vi "S4GUI_003.vi"(7 "Tab ObsEng":enum32{"Obs", "CCD modes", "Guider", "Eng"}(tab)) -> ()   [LabVIEW 2018] (continued)
            n1724 = call-dynamic "Write State Machine.vi"("error in (no error)"=w3191, "State Machine.lvclass"=w3193, "Device in"=w3195) -> ("error out"=w3188:errorcluster, "Device out"=w3189:refnum<class "Channel.lvclass">)  [unwired: 7 in]
            n1725 = call-dynamic "Write Channel.vi"("error in (no error)"=w3188, "Channel.lvclass"=w3189, "Acquisition in"=w3197) -> ("error out"=w3187:errorcluster, "Acquisition out"=w3186:refnum<class "Acquisition.lvclass">)  [unwired: 7 in]
            n1726 = call-dynamic "Write AcquisitionC.vi"("error in (no error)"=w3187, "Acquisition.lvclass"=w3186, "S4ACS_GUI in"=w3199) -> ("error out"=w3157:errorcluster, "S4ACS_GUI out"=w3156:refnum<class "S4GUI.lvclass">)  [unwired: 7 in]
            n1727 = call-dynamic "Read AcquisitionD.vi"("error in (no error)"=w3157, "S4ACS_GUI in"=w3156) -> ("error out"=w3165:errorcluster, "Acquisition.lvclass"=w3163:refnum<class "Acquisition.lvclass">, "S4ACS_GUI out"=w3162:refnum<class "S4GUI.lvclass">)  [unwired: 7 in]
            n1728 = call-dynamic "Read Channel.vi"("error in (no error)"=w3165, "Acquisition in"=w3163) -> ("error out"=w3178:errorcluster, "Channel.lvclass"=w3176:refnum<class "Channel.lvclass">, "Acquisition out"=w3164:refnum<class "Acquisition.lvclass">)  [unwired: 7 in]
            n1729 = call "Write section_name.vi"("error in (no error)"=w3178, "section_name"="CCD_ACS4", "Channel in"=w3176) -> ("error out"=w3179:errorcluster, "Channel out"=w3177:refnum<class "Channel.lvclass">)  [unwired: 7 in]
            n1730 = call-dynamic "load config.vi"("error in (no error)"=w3179, "cfg file name"=w3150, "Channel in"=w3177) -> ("error out"=w3136:errorcluster, "Channel out"=w3134:refnum<class "Channel.lvclass">)  [unwired: 7 in]
            n1731 = call-dynamic "save config.vi"("error in (no error)"=w3136, "file config"="lastsaved.cfg", "Channel in"=w3134) -> ("error out"=w3135:errorcluster, "Channel out"=w3133:refnum<class "Channel.lvclass">)  [unwired: 7 in]
            n1732 = call-dynamic "Read State Machine.vi"("error in (no error)"=w3135, "Device in"=w3133) -> ("error out"=w3169:errorcluster, "State Machine.lvclass"=w3167:refnum<class "State Machine.lvclass">, "Device out"=w3166:refnum<class "Channel.lvclass">)  [unwired: 7 in]
            n1733 = call-dynamic "Write State.vi"("error in (no error)"=w3169, "State"=60, "State Machine in"=w3167) -> ("error out"=w3170:errorcluster, "State Machine out"=w3168:refnum<class "State Machine.lvclass">)  [unwired: 7 in]
            n1734 = call-dynamic "Write State Machine.vi"("error in (no error)"=w3170, "State Machine.lvclass"=w3168, "Device in"=w3166) -> ("error out"=w3173:errorcluster, "Device out"=w3172:refnum<class "Channel.lvclass">)  [unwired: 7 in]
            n1735 = call-dynamic "Write Channel.vi"("error in (no error)"=w3173, "Channel.lvclass"=w3172, "Acquisition in"=w3164) -> ("error out"=w3174:errorcluster, "Acquisition out"=w3175:refnum<class "Acquisition.lvclass">)  [unwired: 7 in]
            n1736 = call-dynamic "Write AcquisitionD.vi"("error in (no error)"=w3174, "Acquisition.lvclass"=w3175, "S4ACS_GUI in"=w3162) -> ("error out"=w3153:errorcluster, "S4ACS_GUI out"=w3155:refnum<class "S4GUI.lvclass">)  [unwired: 7 in]
            n1737 = Unbundle By Name(w3106) -> ("INITIAL_LINE"=w3127:u16, "INITIAL_COLUMN"=w3126:u16, "FINAL_LINE"=w3125:u16, "FINAL_COLUMN"=w3124:u16, "VBIN"=w3123:u16, "HBIN"=w3122:u16, "PREAMP"=w3121:u8, "EM_GAIN"=w3120:u16, "READOUT_RATE"=w3119:u8, "SHUTTER_OPENING_TIME"=w3118:u16, "SHUTTER_CLOSING_TIME"=w3117:u16, "VERTICAL_SHIFT_SPEED"=w3107:u8, "READ_MODE"=w3116:u8, "VERTICAL_CLOCK_VOLTAGE"=w3115:u8, "AD_CHANNEL"=w3114:u32, "SHUTTER_MODE"=w3113:u8, "SHUTTER_TTL"=w3112:u8, "TRIGGER_MODE"=w3111:u8, "FRAME_TRANSFER"=w3110:bool, "ACQUISITION_MODE"=w3109:u8, "EM_MODE"=w3108:u8)
            n1738 = call "Write cfg file.vi"("error in (no error)"=w3153, "cfg file"=w3150, "S4ACS_GUI in"=w3155) -> ("error out"=w3152:errorcluster, "S4ACS_GUI out"=w3154:refnum<class "S4GUI.lvclass">)  [unwired: 7 in]
            n1739 = local read "Input Cluster"() -> (w3129:T8)
            n1740 = Bundle By Name(cluster=w3129, "Parameters.Image \nInitial Line"=w3127, "Parameters.Image\nInitial Column"=w3126, "Parameters.Image\nFinal Line"=w3125, "Parameters.Image\nFInal Column"=w3124, "Parameters.Vertical\nBinning"=w3123, "Parameters.Horizontal\nBinning"=w3122, "Parameters.Pre-amplification\nGain"=w3121, "Parameters.CCD\nEM Gain"=w3120, "Parameters.Readout\nRate"=w3119, "Parameters.Shutter\nOpenning Time"=w3118, "Parameters.Shutter\nClosing Time"=w3117, "Parameters.Vertical\nShift Speed"=w3107, "Parameters.Read\nMode"=w3116, "Parameters.Vertical\nClock Voltage"=w3115, "Parameters.A/D \nChannel"=w3114, "Parameters.Shutter\nMode"=w3113, "Parameters.Shutter\nTTL"=w3112, "Parameters.Trigger\nMode"=w3111, "Parameters.Frame\nTransfer"=w3110, "Parameters.Acquisition\nMode"=w3109, "Parameters.CCD \nEM Mode"=w3108) -> (w3128:T8)
            n1741 = local write "Input Cluster"(w3128) -> ()
          }
          frame True {
          }
        }
      }
      event "Save As Button": Value Change {
        n1742 = event-data() -> ()  [unwired: 1 in, 6 out]
        n1743 = disable-structure shown="Enabled" {
          disable-tunnel: [w3254 w3266] -> w3243
          disable-tunnel: w3242 -> [w3253 _]
          disable-tunnel: [w3247 w3264] -> w3241
          frame Disabled {
            n1744 = String To Path(string="C:\\Users\\observer\\sparc4\\s4gui\\Config" ("default name")) -> (path=w3249:path)
            n1745 = call "File Dialog2"("start path"=w3249, "prompt"="Select file...", "button label"="Save", "default name"="lastsaved.cfg", "error in"=w3253, "pattern (all files)"="*.cfg") -> ("selected path"=w3248:path, "cancelled"=w3254:bool, "error out"=→"error out 3":errorcluster)  [unwired: 6 in, 1 out]
            n1746 = Strip Path(path=w3248) -> (name=w3247:string)  [unwired: 1 out]
          }
          frame Enabled {
            w3268 = ".cfg" ("regular expression")
            n1747 = Match Pattern(string="savefile", regular expression=w3268) -> (before substring=w3263:string, match substring=w3267:string)  [unwired: 1 in, 2 out]
            n1748 = String Length(string=w3263) -> (length=w3262:i32)
            n1749 = Equal?(x=w3267, y=w3268) -> (x = y?=w3258:bool)
            n1750 = Less?(x=w3262, y=20) -> (x < y?=w3259:bool)
            n1751 = And(x=w3259, y=w3258) -> (x .and. y?=w3260:bool)
            n1752 = case shown="False" w3260 {
              tunnel: w3263 -> [_ w3281]
              tunnel: w3267 -> [_ w3280]
              tunnel: [TRUE ("cancelled") FALSE ("cancelled")] -> w3266
              tunnel: [w3271 w3279] -> w3264
              tunnel: [w3271 w3279] -> w3265
              frame False {
                w3271 = "lastsaved.cfg" ("savefile")
                n1753 = One Button Dialog(message="Invalid file name!\nFile name length must be less than 20 characters\nand must contain .cfg ending." ("savefile")) -> ()  [unwired: 1 in, 1 out]
              }
              frame True {
                n1754 = call <vilib>:"Trim Whitespace.vi"("string"=w3281) -> ("trimmed string"=w3278:string)  [unwired: 1 in]
                n1755 = call <vilib>:"Space Constant.vi"() -> ("String"=w3276:string)
                n1756 = To Lower Case(string=w3278) -> (all lower case string=w3274:string)
                n1757 = Search and Replace String(replace all?=TRUE ("replace all? (F)"), input string=w3274, search string=w3276, replace string="" ("replace string (\"\")")) -> (result string=w3273:string)  [unwired: 4 in, 3 out]
                n1758 = Concatenate Strings(w3273, w3280) -> (w3279:string)
              }
            }
            n1759 = local write "savefile"(w3265) -> ()
          }
        }
        n1760 = case shown="False" w3243 {
          tunnel: w3246 -> [w3347 w3349]
          tunnel: [w3295 w3349] -> w3245
          tunnel: [w3293 w3348] -> w3244
          tunnel: w3242 -> [w3292 w3348]
          tunnel: w3241 -> [w3291 _]
          frame False {
            n1761 = call-dynamic "Read AcquisitionA.vi"("error in (no error)"=w3292, "S4ACS_GUI in"=w3347) -> ("error out"=w3343:errorcluster, "Acquisition.lvclass"=w3345:refnum<class "Acquisition.lvclass">, "S4ACS_GUI out"=w3346:refnum<class "S4GUI.lvclass">)  [unwired: 7 in]
            n1762 = call-dynamic "Read Channel.vi"("error in (no error)"=w3343, "Acquisition in"=w3345) -> ("error out"=w3338:errorcluster, "Channel.lvclass"=w3340:refnum<class "Channel.lvclass">, "Acquisition out"=w3344:refnum<class "Acquisition.lvclass">)  [unwired: 7 in]
            n1763 = call "Write section_name.vi"("error in (no error)"=w3338, "section_name"="CCD_ACS1", "Channel in"=w3340) -> ("error out"=w3337:errorcluster, "Channel out"=w3339:refnum<class "Channel.lvclass">)  [unwired: 7 in]
            n1764 = call-dynamic "save config.vi"("error in (no error)"=w3337, "file config"=w3291, "Channel in"=w3339) -> ("error out"=w3289:errorcluster, "Channel out"=w3290:refnum<class "Channel.lvclass">)  [unwired: 7 in]
            n1765 = call-dynamic "Write Channel.vi"("error in (no error)"=w3289, "Channel.lvclass"=w3290, "Acquisition in"=w3344) -> ("error out"=w3342:errorcluster, "Acquisition out"=w3341:refnum<class "Acquisition.lvclass">)  [unwired: 7 in]
            n1766 = call-dynamic "Write AcquisitionA.vi"("error in (no error)"=w3342, "Acquisition.lvclass"=w3341, "S4ACS_GUI in"=w3346) -> ("error out"=w3302:errorcluster, "S4ACS_GUI out"=w3301:refnum<class "S4GUI.lvclass">)  [unwired: 7 in]
            n1767 = call "Read AcquisitionB.vi"("error in (no error)"=w3302, "S4ACS_GUI in"=w3301) -> ("error out"=w3328:errorcluster, "Acquisition.lvclass"=w3326:refnum<class "Acquisition.lvclass">, "S4ACS_GUI out"=w3325:refnum<class "S4GUI.lvclass">)  [unwired: 7 in]
            n1768 = call-dynamic "Read Channel.vi"("error in (no error)"=w3328, "Acquisition in"=w3326) -> ("error out"=w3333:errorcluster, "Channel.lvclass"=w3331:refnum<class "Channel.lvclass">, "Acquisition out"=w3327:refnum<class "Acquisition.lvclass">)  [unwired: 7 in]
            n1769 = call "Write section_name.vi"("error in (no error)"=w3333, "section_name"="CCD_ACS2", "Channel in"=w3331) -> ("error out"=w3334:errorcluster, "Channel out"=w3332:refnum<class "Channel.lvclass">)  [unwired: 7 in]
            n1770 = call-dynamic "save config.vi"("error in (no error)"=w3334, "file config"=w3291, "Channel in"=w3332) -> ("error out"=w3283:errorcluster, "Channel out"=w3284:refnum<class "Channel.lvclass">)  [unwired: 7 in]
            n1771 = call-dynamic "Write Channel.vi"("error in (no error)"=w3283, "Channel.lvclass"=w3284, "Acquisition in"=w3327) -> ("error out"=w3329:errorcluster, "Acquisition out"=w3330:refnum<class "Acquisition.lvclass">)  [unwired: 7 in]
            n1772 = call "Write AcquisitionB.vi"("error in (no error)"=w3329, "Acquisition.lvclass"=w3330, "S4ACS_GUI in"=w3325) -> ("error out"=w3300:errorcluster, "S4ACS_GUI out"=w3299:refnum<class "S4GUI.lvclass">)  [unwired: 7 in]
            n1773 = call-dynamic "Read AcquisitionC.vi"("error in (no error)"=w3300, "S4ACS_GUI in"=w3299) -> ("error out"=w3321:errorcluster, "Acquisition.lvclass"=w3323:refnum<class "Acquisition.lvclass">, "S4ACS_GUI out"=w3324:refnum<class "S4GUI.lvclass">)  [unwired: 7 in]
            n1774 = call-dynamic "Read Channel.vi"("error in (no error)"=w3321, "Acquisition in"=w3323) -> ("error out"=w3316:errorcluster, "Channel.lvclass"=w3318:refnum<class "Channel.lvclass">, "Acquisition out"=w3322:refnum<class "Acquisition.lvclass">)  [unwired: 7 in]
            n1775 = call "Write section_name.vi"("error in (no error)"=w3316, "section_name"="CCD_ACS3", "Channel in"=w3318) -> ("error out"=w3315:errorcluster, "Channel out"=w3317:refnum<class "Channel.lvclass">)  [unwired: 7 in]
            n1776 = call-dynamic "save config.vi"("error in (no error)"=w3315, "file config"=w3291, "Channel in"=w3317) -> ("error out"=w3285:errorcluster, "Channel out"=w3286:refnum<class "Channel.lvclass">)  [unwired: 7 in]
            n1777 = call-dynamic "Write Channel.vi"("error in (no error)"=w3285, "Channel.lvclass"=w3286, "Acquisition in"=w3322) -> ("error out"=w3320:errorcluster, "Acquisition out"=w3319:refnum<class "Acquisition.lvclass">)  [unwired: 7 in]
            n1778 = call-dynamic "Write AcquisitionC.vi"("error in (no error)"=w3320, "Acquisition.lvclass"=w3319, "S4ACS_GUI in"=w3324) -> ("error out"=w3298:errorcluster, "S4ACS_GUI out"=w3297:refnum<class "S4GUI.lvclass">)  [unwired: 7 in]
            n1779 = call-dynamic "Read AcquisitionD.vi"("error in (no error)"=w3298, "S4ACS_GUI in"=w3297) -> ("error out"=w3306:errorcluster, "Acquisition.lvclass"=w3304:refnum<class "Acquisition.lvclass">, "S4ACS_GUI out"=w3303:refnum<class "S4GUI.lvclass">)  [unwired: 7 in]
            n1780 = call-dynamic "Read Channel.vi"("error in (no error)"=w3306, "Acquisition in"=w3304) -> ("error out"=w3311:errorcluster, "Channel.lvclass"=w3309:refnum<class "Channel.lvclass">, "Acquisition out"=w3305:refnum<class "Acquisition.lvclass">)  [unwired: 7 in]
            n1781 = call "Write section_name.vi"("error in (no error)"=w3311, "section_name"="CCD_ACS4", "Channel in"=w3309) -> ("error out"=w3312:errorcluster, "Channel out"=w3310:refnum<class "Channel.lvclass">)  [unwired: 7 in]
            n1782 = call-dynamic "save config.vi"("error in (no error)"=w3312, "file config"=w3291, "Channel in"=w3310) -> ("error out"=w3287:errorcluster, "Channel out"=w3288:refnum<class "Channel.lvclass">)  [unwired: 7 in]
            n1783 = call-dynamic "Write Channel.vi"("error in (no error)"=w3287, "Channel.lvclass"=w3288, "Acquisition in"=w3305) -> ("error out"=w3307:errorcluster, "Acquisition out"=w3308:refnum<class "Acquisition.lvclass">)  [unwired: 7 in]
            n1784 = call-dynamic "Write AcquisitionD.vi"("error in (no error)"=w3307, "Acquisition.lvclass"=w3308, "S4ACS_GUI in"=w3303) -> ("error out"=w3294:errorcluster, "S4ACS_GUI out"=w3296:refnum<class "S4GUI.lvclass">)  [unwired: 7 in]
            n1785 = call "Write cfg file.vi"("error in (no error)"=w3294, "cfg file"=w3291, "S4ACS_GUI in"=w3296) -> ("error out"=w3293:errorcluster, "S4ACS_GUI out"=w3295:refnum<class "S4GUI.lvclass">)  [unwired: 7 in]
          }
          frame True {
          }
        }
      }
      event "Load Default Button": Value Change {
        w3394 = "default.cfg" ("cfg file name")
        n1786 = event-data() -> ()  [unwired: 1 in, 6 out]
        n1787 = call-dynamic "Read AcquisitionA.vi"("error in (no error)"=w3484, "S4ACS_GUI in"=w3485) -> ("error out"=w3480:errorcluster, "Acquisition.lvclass"=w3482:refnum<class "Acquisition.lvclass">, "S4ACS_GUI out"=w3483:refnum<class "S4GUI.lvclass">)  [unwired: 7 in]
        n1788 = call-dynamic "Read Channel.vi"("error in (no error)"=w3480, "Acquisition in"=w3482) -> ("error out"=w3467:errorcluster, "Channel.lvclass"=w3469:refnum<class "Channel.lvclass">, "Acquisition out"=w3481:refnum<class "Acquisition.lvclass">)  [unwired: 7 in]
        n1789 = call "Write section_name.vi"("error in (no error)"=w3467, "section_name"="CCD_ACS1", "Channel in"=w3469) -> ("error out"=w3466:errorcluster, "Channel out"=w3468:refnum<class "Channel.lvclass">)  [unwired: 7 in]
        n1790 = call-dynamic "load config.vi"("error in (no error)"=w3466, "cfg file name"=w3394, "Channel in"=w3468) -> ("error out"=w3392:errorcluster, "Channel out"=w3393:refnum<class "Channel.lvclass">)  [unwired: 7 in]
        n1791 = call-dynamic "save config.vi"("error in (no error)"=w3392, "file config"="lastsaved.cfg", "Channel in"=w3393) -> ("error out"=w3351:errorcluster, "Channel out"=w3352:refnum<class "Channel.lvclass">)  [unwired: 7 in]
        n1792 = call-dynamic "Read target cluster.vi"("error in (no error)"=w3351, "Channel in"=w3352) -> ("target cluster"=w3350:T31)  [unwired: 7 in, 2 out]
        n1793 = call-dynamic "Read State Machine.vi"("error in (no error)"=w3351, "Device in"=w3352) -> ("error out"=w3476:errorcluster, "State Machine.lvclass"=w3478:refnum<class "State Machine.lvclass">, "Device out"=w3479:refnum<class "Channel.lvclass">)  [unwired: 7 in]
        n1794 = call-dynamic "Write State.vi"("error in (no error)"=w3476, "State"=60, "State Machine in"=w3478) -> ("error out"=w3475:errorcluster, "State Machine out"=w3477:refnum<class "State Machine.lvclass">)  [unwired: 7 in]
        n1795 = call-dynamic "Write State Machine.vi"("error in (no error)"=w3475, "State Machine.lvclass"=w3477, "Device in"=w3479) -> ("error out"=w3472:errorcluster, "Device out"=w3473:refnum<class "Channel.lvclass">)  [unwired: 7 in]
        n1796 = call-dynamic "Write Channel.vi"("error in (no error)"=w3472, "Channel.lvclass"=w3473, "Acquisition in"=w3481) -> ("error out"=w3471:errorcluster, "Acquisition out"=w3470:refnum<class "Acquisition.lvclass">)  [unwired: 7 in]
        n1797 = call-dynamic "Write AcquisitionA.vi"("error in (no error)"=w3471, "Acquisition.lvclass"=w3470, "S4ACS_GUI in"=w3483) -> ("error out"=w3404:errorcluster, "S4ACS_GUI out"=w3403:refnum<class "S4GUI.lvclass">)  [unwired: 7 in]
        n1798 = call "Read AcquisitionB.vi"("error in (no error)"=w3404, "S4ACS_GUI in"=w3403) -> ("error out"=w3448:errorcluster, "Acquisition.lvclass"=w3446:refnum<class "Acquisition.lvclass">, "S4ACS_GUI out"=w3445:refnum<class "S4GUI.lvclass">)  [unwired: 7 in]
        n1799 = call-dynamic "Read Channel.vi"("error in (no error)"=w3448, "Acquisition in"=w3446) -> ("error out"=w3462:errorcluster, "Channel.lvclass"=w3460:refnum<class "Channel.lvclass">, "Acquisition out"=w3447:refnum<class "Acquisition.lvclass">)  [unwired: 7 in]
        n1800 = call "Write section_name.vi"("error in (no error)"=w3462, "section_name"="CCD_ACS2", "Channel in"=w3460) -> ("error out"=w3463:errorcluster, "Channel out"=w3461:refnum<class "Channel.lvclass">)  [unwired: 7 in]
        n1801 = call-dynamic "load config.vi"("error in (no error)"=w3463, "cfg file name"="default.cfg", "Channel in"=w3461) -> ("error out"=w3389:errorcluster, "Channel out"=w3387:refnum<class "Channel.lvclass">)  [unwired: 7 in]
        n1802 = call-dynamic "save config.vi"("error in (no error)"=w3389, "file config"="lastsaved.cfg", "Channel in"=w3387) -> ("error out"=w3388:errorcluster, "Channel out"=w3386:refnum<class "Channel.lvclass">)  [unwired: 7 in]
        n1803 = call-dynamic "Read State Machine.vi"("error in (no error)"=w3388, "Device in"=w3386) -> ("error out"=w3452:errorcluster, "State Machine.lvclass"=w3450:refnum<class "State Machine.lvclass">, "Device out"=w3449:refnum<class "Channel.lvclass">)  [unwired: 7 in]
        n1804 = call-dynamic "Write State.vi"("error in (no error)"=w3452, "State"=60, "State Machine in"=w3450) -> ("error out"=w3453:errorcluster, "State Machine out"=w3451:refnum<class "State Machine.lvclass">)  [unwired: 7 in]
        n1805 = call-dynamic "Write State Machine.vi"("error in (no error)"=w3453, "State Machine.lvclass"=w3451, "Device in"=w3449) -> ("error out"=w3456:errorcluster, "Device out"=w3455:refnum<class "Channel.lvclass">)  [unwired: 7 in]
        n1806 = call-dynamic "Write Channel.vi"("error in (no error)"=w3456, "Channel.lvclass"=w3455, "Acquisition in"=w3447) -> ("error out"=w3457:errorcluster, "Acquisition out"=w3458:refnum<class "Acquisition.lvclass">)  [unwired: 7 in]
        n1807 = call "Write AcquisitionB.vi"("error in (no error)"=w3457, "Acquisition.lvclass"=w3458, "S4ACS_GUI in"=w3445) -> ("error out"=w3402:errorcluster, "S4ACS_GUI out"=w3401:refnum<class "S4GUI.lvclass">)  [unwired: 7 in]
        n1808 = call-dynamic "Read AcquisitionC.vi"("error in (no error)"=w3402, "S4ACS_GUI in"=w3401) -> ("error out"=w3441:errorcluster, "Acquisition.lvclass"=w3443:refnum<class "Acquisition.lvclass">, "S4ACS_GUI out"=w3444:refnum<class "S4GUI.lvclass">)  [unwired: 7 in]
        n1809 = call-dynamic "Read Channel.vi"("error in (no error)"=w3441, "Acquisition in"=w3443) -> ("error out"=w3427:errorcluster, "Channel.lvclass"=w3429:refnum<class "Channel.lvclass">, "Acquisition out"=w3442:refnum<class "Acquisition.lvclass">)  [unwired: 7 in]
        n1810 = call "Write section_name.vi"("error in (no error)"=w3427, "section_name"="CCD_ACS3", "Channel in"=w3429) -> ("error out"=w3426:errorcluster, "Channel out"=w3428:refnum<class "Channel.lvclass">)  [unwired: 7 in]
        n1811 = call-dynamic "load config.vi"("error in (no error)"=w3426, "cfg file name"="default.cfg", "Channel in"=w3428) -> ("error out"=w3383:errorcluster, "Channel out"=w3384:refnum<class "Channel.lvclass">)  [unwired: 7 in]
        n1812 = call-dynamic "save config.vi"("error in (no error)"=w3383, "file config"="lastsaved.cfg", "Channel in"=w3384) -> ("error out"=w3381:errorcluster, "Channel out"=w3382:refnum<class "Channel.lvclass">)  [unwired: 7 in]
        n1813 = call-dynamic "Read State Machine.vi"("error in (no error)"=w3381, "Device in"=w3382) -> ("error out"=w3437:errorcluster, "State Machine.lvclass"=w3439:refnum<class "State Machine.lvclass">, "Device out"=w3440:refnum<class "Channel.lvclass">)  [unwired: 7 in]
        n1814 = call-dynamic "Write State.vi"("error in (no error)"=w3437, "State"=60, "State Machine in"=w3439) -> ("error out"=w3436:errorcluster, "State Machine out"=w3438:refnum<class "State Machine.lvclass">)  [unwired: 7 in]
        n1815 = call-dynamic "Write State Machine.vi"("error in (no error)"=w3436, "State Machine.lvclass"=w3438, "Device in"=w3440) -> ("error out"=w3433:errorcluster, "Device out"=w3434:refnum<class "Channel.lvclass">)  [unwired: 7 in]
        n1816 = call-dynamic "Write Channel.vi"("error in (no error)"=w3433, "Channel.lvclass"=w3434, "Acquisition in"=w3442) -> ("error out"=w3432:errorcluster, "Acquisition out"=w3431:refnum<class "Acquisition.lvclass">)  [unwired: 7 in]
        n1817 = call-dynamic "Write AcquisitionC.vi"("error in (no error)"=w3432, "Acquisition.lvclass"=w3431, "S4ACS_GUI in"=w3444) -> ("error out"=w3400:errorcluster, "S4ACS_GUI out"=w3399:refnum<class "S4GUI.lvclass">)  [unwired: 7 in]
        n1818 = call-dynamic "Read AcquisitionD.vi"("error in (no error)"=w3400, "S4ACS_GUI in"=w3399) -> ("error out"=w3408:errorcluster, "Acquisition.lvclass"=w3406:refnum<class "Acquisition.lvclass">, "S4ACS_GUI out"=w3405:refnum<class "S4GUI.lvclass">)  [unwired: 7 in]
        n1819 = call-dynamic "Read Channel.vi"("error in (no error)"=w3408, "Acquisition in"=w3406) -> ("error out"=w3422:errorcluster, "Channel.lvclass"=w3420:refnum<class "Channel.lvclass">, "Acquisition out"=w3407:refnum<class "Acquisition.lvclass">)  [unwired: 7 in]
        n1820 = call "Write section_name.vi"("error in (no error)"=w3422, "section_name"="CCD_ACS4", "Channel in"=w3420) -> ("error out"=w3423:errorcluster, "Channel out"=w3421:refnum<class "Channel.lvclass">)  [unwired: 7 in]
        n1821 = call-dynamic "load config.vi"("error in (no error)"=w3423, "cfg file name"="default.cfg", "Channel in"=w3421) -> ("error out"=w3379:errorcluster, "Channel out"=w3378:refnum<class "Channel.lvclass">)  [unwired: 7 in]
        n1822 = call-dynamic "save config.vi"("error in (no error)"=w3379, "file config"="lastsaved.cfg", "Channel in"=w3378) -> ("error out"=w3376:errorcluster, "Channel out"=w3377:refnum<class "Channel.lvclass">)  [unwired: 7 in]
        n1823 = call-dynamic "Read State Machine.vi"("error in (no error)"=w3376, "Device in"=w3377) -> ("error out"=w3412:errorcluster, "State Machine.lvclass"=w3410:refnum<class "State Machine.lvclass">, "Device out"=w3409:refnum<class "Channel.lvclass">)  [unwired: 7 in]
        n1824 = call-dynamic "Write State.vi"("error in (no error)"=w3412, "State"=60, "State Machine in"=w3410) -> ("error out"=w3413:errorcluster, "State Machine out"=w3411:refnum<class "State Machine.lvclass">)  [unwired: 7 in]
        n1825 = call-dynamic "Write State Machine.vi"("error in (no error)"=w3413, "State Machine.lvclass"=w3411, "Device in"=w3409) -> ("error out"=w3416:errorcluster, "Device out"=w3415:refnum<class "Channel.lvclass">)  [unwired: 7 in]
        n1826 = call-dynamic "Write Channel.vi"("error in (no error)"=w3416, "Channel.lvclass"=w3415, "Acquisition in"=w3407) -> ("error out"=w3417:errorcluster, "Acquisition out"=w3418:refnum<class "Acquisition.lvclass">)  [unwired: 7 in]
        n1827 = call-dynamic "Write AcquisitionD.vi"("error in (no error)"=w3417, "Acquisition.lvclass"=w3418, "S4ACS_GUI in"=w3405) -> ("error out"=w3396:errorcluster, "S4ACS_GUI out"=w3398:refnum<class "S4GUI.lvclass">)  [unwired: 7 in]
        n1828 = Unbundle By Name(w3350) -> ("INITIAL_LINE"=w3355:u16, "INITIAL_COLUMN"=w3356:u16, "FINAL_LINE"=w3357:u16, "FINAL_COLUMN"=w3358:u16, "VBIN"=w3359:u16, "HBIN"=w3360:u16, "PREAMP"=w3361:u8, "EM_GAIN"=w3362:u16, "READOUT_RATE"=w3363:u8, "SHUTTER_OPENING_TIME"=w3364:u16, "SHUTTER_CLOSING_TIME"=w3365:u16, "VERTICAL_SHIFT_SPEED"=w3375:u8, "READ_MODE"=w3366:u8, "VERTICAL_CLOCK_VOLTAGE"=w3367:u8, "AD_CHANNEL"=w3368:u32, "SHUTTER_MODE"=w3369:u8, "SHUTTER_TTL"=w3370:u8, "TRIGGER_MODE"=w3371:u8, "FRAME_TRANSFER"=w3372:bool, "ACQUISITION_MODE"=w3373:u8, "EM_MODE"=w3374:u8)
        n1829 = call "Write cfg file.vi"("error in (no error)"=w3396, "cfg file"=w3394, "S4ACS_GUI in"=w3398) -> ("error out"=w3395:errorcluster, "S4ACS_GUI out"=w3397:refnum<class "S4GUI.lvclass">)  [unwired: 7 in]
        n1830 = local read "Input Cluster"() -> (w3353:T8)
        n1831 = Bundle By Name(cluster=w3353, "Parameters.Image \nInitial Line"=w3355, "Parameters.Image\nInitial Column"=w3356, "Parameters.Image\nFinal Line"=w3357, "Parameters.Image\nFInal Column"=w3358, "Parameters.Vertical\nBinning"=w3359, "Parameters.Horizontal\nBinning"=w3360, "Parameters.Pre-amplification\nGain"=w3361, "Parameters.CCD\nEM Gain"=w3362, "Parameters.Readout\nRate"=w3363, "Parameters.Shutter\nOpenning Time"=w3364, "Parameters.Shutter\nClosing Time"=w3365, "Parameters.Vertical\nShift Speed"=w3375, "Parameters.Read\nMode"=w3366, "Parameters.Vertical\nClock Voltage"=w3367, "Parameters.A/D \nChannel"=w3368, "Parameters.Shutter\nMode"=w3369, "Parameters.Shutter\nTTL"=w3370, "Parameters.Trigger\nMode"=w3371, "Parameters.Frame\nTransfer"=w3372, "Parameters.Acquisition\nMode"=w3373, "Parameters.CCD \nEM Mode"=w3374) -> (w3354:T8)
        n1832 = local write "Input Cluster"(w3354) -> ()
      }
      event "Restore Default ch2": Value Change {
        n1833 = event-data() -> ()  [unwired: 1 in, 6 out]
        n1834 = call "Read AcquisitionB.vi"("error in (no error)"=w3516, "S4ACS_GUI in"=w3517) -> ("error out"=w3512:errorcluster, "Acquisition.lvclass"=w3514:refnum<class "Acquisition.lvclass">, "S4ACS_GUI out"=w3515:refnum<class "S4GUI.lvclass">)  [unwired: 7 in]
        n1835 = call-dynamic "Read Channel.vi"("error in (no error)"=w3512, "Acquisition in"=w3514) -> ("error out"=w3499:errorcluster, "Channel.lvclass"=w3501:refnum<class "Channel.lvclass">, "Acquisition out"=w3513:refnum<class "Acquisition.lvclass">)  [unwired: 7 in]
        n1836 = call "Write section_name.vi"("error in (no error)"=w3499, "section_name"="CCD_ACS2", "Channel in"=w3501) -> ("error out"=w3498:errorcluster, "Channel out"=w3500:refnum<class "Channel.lvclass">)  [unwired: 7 in]
        n1837 = call-dynamic "load config.vi"("error in (no error)"=w3498, "cfg file name"="default.cfg", "Channel in"=w3500) -> ("error out"=w3496:errorcluster, "Channel out"=w3497:refnum<class "Channel.lvclass">)  [unwired: 7 in]
        n1838 = call-dynamic "Read State Machine.vi"("error in (no error)"=w3496, "Device in"=w3497) -> ("error out"=w3508:errorcluster, "State Machine.lvclass"=w3510:refnum<class "State Machine.lvclass">, "Device out"=w3511:refnum<class "Channel.lvclass">)  [unwired: 7 in]
        n1839 = call-dynamic "Write State.vi"("error in (no error)"=w3508, "State"=60, "State Machine in"=w3510) -> ("error out"=w3507:errorcluster, "State Machine out"=w3509:refnum<class "State Machine.lvclass">)  [unwired: 7 in]
        n1840 = call-dynamic "Write State Machine.vi"("error in (no error)"=w3507, "State Machine.lvclass"=w3509, "Device in"=w3511) -> ("error out"=w3492:errorcluster, "Device out"=w3489:refnum<class "Channel.lvclass">)  [unwired: 7 in]
        n1841 = call "Write section_name.vi"("error in (no error)"=w3492, "section_name"="CCD_ACS2", "Channel in"=w3489) -> ("error out"=w3493:errorcluster, "Channel out"=w3488:refnum<class "Channel.lvclass">)  [unwired: 7 in]
        n1842 = call-dynamic "save config.vi"("error in (no error)"=w3493, "file config"="lastsaved.cfg", "Channel in"=w3488) -> ("error out"=w3491:errorcluster, "Channel out"=w3487:refnum<class "Channel.lvclass">)  [unwired: 7 in]
        n1843 = call-dynamic "Write Channel.vi"("error in (no error)"=w3491, "Channel.lvclass"=w3487, "Acquisition in"=w3513) -> ("error out"=w3505:errorcluster, "Acquisition out"=w3504:refnum<class "Acquisition.lvclass">)  [unwired: 7 in]
        n1844 = call "Write AcquisitionB.vi"("error in (no error)"=w3505, "Acquisition.lvclass"=w3504, "S4ACS_GUI in"=w3515) -> ("error out"=w3503:errorcluster, "S4ACS_GUI out"=w3494:refnum<class "S4GUI.lvclass">)  [unwired: 7 in]
      }
      event "Restore Default ch3": Value Change {
        n1845 = event-data() -> ()  [unwired: 1 in, 6 out]
        n1846 = call-dynamic "Read AcquisitionC.vi"("error in (no error)"=w3548, "S4ACS_GUI in"=w3549) -> ("error out"=w3544:errorcluster, "Acquisition.lvclass"=w3546:refnum<class "Acquisition.lvclass">, "S4ACS_GUI out"=w3547:refnum<class "S4GUI.lvclass">)  [unwired: 7 in]
        n1847 = call-dynamic "Read Channel.vi"("error in (no error)"=w3544, "Acquisition in"=w3546) -> ("error out"=w3531:errorcluster, "Channel.lvclass"=w3533:refnum<class "Channel.lvclass">, "Acquisition out"=w3545:refnum<class "Acquisition.lvclass">)  [unwired: 7 in]
        n1848 = call "Write section_name.vi"("error in (no error)"=w3531, "section_name"="CCD_ACS3", "Channel in"=w3533) -> ("error out"=w3530:errorcluster, "Channel out"=w3532:refnum<class "Channel.lvclass">)  [unwired: 7 in]
        n1849 = call-dynamic "load config.vi"("error in (no error)"=w3530, "cfg file name"="default.cfg", "Channel in"=w3532) -> ("error out"=w3528:errorcluster, "Channel out"=w3529:refnum<class "Channel.lvclass">)  [unwired: 7 in]
        n1850 = call-dynamic "Read State Machine.vi"("error in (no error)"=w3528, "Device in"=w3529) -> ("error out"=w3540:errorcluster, "State Machine.lvclass"=w3542:refnum<class "State Machine.lvclass">, "Device out"=w3543:refnum<class "Channel.lvclass">)  [unwired: 7 in]
        n1851 = call-dynamic "Write State.vi"("error in (no error)"=w3540, "State"=60, "State Machine in"=w3542) -> ("error out"=w3539:errorcluster, "State Machine out"=w3541:refnum<class "State Machine.lvclass">)  [unwired: 7 in]
        n1852 = call-dynamic "Write State Machine.vi"("error in (no error)"=w3539, "State Machine.lvclass"=w3541, "Device in"=w3543) -> ("error out"=w3519:errorcluster, "Device out"=w3521:refnum<class "Channel.lvclass">)  [unwired: 7 in]
        n1853 = call "Write section_name.vi"("error in (no error)"=w3519, "section_name"="CCD_ACS3", "Channel in"=w3521) -> ("error out"=w3525:errorcluster, "Channel out"=w3520:refnum<class "Channel.lvclass">)  [unwired: 7 in]
        n1854 = call-dynamic "save config.vi"("error in (no error)"=w3525, "file config"="lastsaved.cfg", "Channel in"=w3520) -> ("error out"=w3518:errorcluster, "Channel out"=w3522:refnum<class "Channel.lvclass">)  [unwired: 7 in]
        n1855 = call-dynamic "Write Channel.vi"("error in (no error)"=w3518, "Channel.lvclass"=w3522, "Acquisition in"=w3545) -> ("error out"=w3537:errorcluster, "Acquisition out"=w3536:refnum<class "Acquisition.lvclass">)  [unwired: 7 in]
        n1856 = call-dynamic "Write AcquisitionC.vi"("error in (no error)"=w3537, "Acquisition.lvclass"=w3536, "S4ACS_GUI in"=w3547) -> ("error out"=w3535:errorcluster, "S4ACS_GUI out"=w3526:refnum<class "S4GUI.lvclass">)  [unwired: 7 in]
      }
      event "Restore Default ch4": Value Change {
        n1857 = event-data() -> ()  [unwired: 1 in, 6 out]
        n1858 = call-dynamic "Read AcquisitionD.vi"("error in (no error)"=w3580, "S4ACS_GUI in"=w3581) -> ("error out"=w3576:errorcluster, "Acquisition.lvclass"=w3578:refnum<class "Acquisition.lvclass">, "S4ACS_GUI out"=w3579:refnum<class "S4GUI.lvclass">)  [unwired: 7 in]
        n1859 = call-dynamic "Read Channel.vi"("error in (no error)"=w3576, "Acquisition in"=w3578) -> ("error out"=w3563:errorcluster, "Channel.lvclass"=w3565:refnum<class "Channel.lvclass">, "Acquisition out"=w3577:refnum<class "Acquisition.lvclass">)  [unwired: 7 in]
        n1860 = call "Write section_name.vi"("error in (no error)"=w3563, "section_name"="CCD_ACS4", "Channel in"=w3565) -> ("error out"=w3562:errorcluster, "Channel out"=w3564:refnum<class "Channel.lvclass">)  [unwired: 7 in]
        n1861 = call-dynamic "load config.vi"("error in (no error)"=w3562, "cfg file name"="default.cfg", "Channel in"=w3564) -> ("error out"=w3560:errorcluster, "Channel out"=w3561:refnum<class "Channel.lvclass">)  [unwired: 7 in]
        n1862 = call-dynamic "Read State Machine.vi"("error in (no error)"=w3560, "Device in"=w3561) -> ("error out"=w3572:errorcluster, "State Machine.lvclass"=w3574:refnum<class "State Machine.lvclass">, "Device out"=w3575:refnum<class "Channel.lvclass">)  [unwired: 7 in]
        n1863 = call-dynamic "Write State.vi"("error in (no error)"=w3572, "State"=60, "State Machine in"=w3574) -> ("error out"=w3571:errorcluster, "State Machine out"=w3573:refnum<class "State Machine.lvclass">)  [unwired: 7 in]
        n1864 = call-dynamic "Write State Machine.vi"("error in (no error)"=w3571, "State Machine.lvclass"=w3573, "Device in"=w3575) -> ("error out"=w3551:errorcluster, "Device out"=w3554:refnum<class "Channel.lvclass">)  [unwired: 7 in]
        n1865 = call "Write section_name.vi"("error in (no error)"=w3551, "section_name"="CCD_ACS4", "Channel in"=w3554) -> ("error out"=w3557:errorcluster, "Channel out"=w3553:refnum<class "Channel.lvclass">)  [unwired: 7 in]
        n1866 = call-dynamic "save config.vi"("error in (no error)"=w3557, "file config"="lastsaved.cfg", "Channel in"=w3553) -> ("error out"=w3550:errorcluster, "Channel out"=w3552:refnum<class "Channel.lvclass">)  [unwired: 7 in]
        n1867 = call-dynamic "Write Channel.vi"("error in (no error)"=w3550, "Channel.lvclass"=w3552, "Acquisition in"=w3577) -> ("error out"=w3569:errorcluster, "Acquisition out"=w3568:refnum<class "Acquisition.lvclass">)  [unwired: 7 in]
        n1868 = call-dynamic "Write AcquisitionD.vi"("error in (no error)"=w3569, "Acquisition.lvclass"=w3568, "S4ACS_GUI in"=w3579) -> ("error out"=w3567:errorcluster, "S4ACS_GUI out"=w3558:refnum<class "S4GUI.lvclass">)  [unwired: 7 in]
      }
      event "Copy to Input ch1": Value Change {
        w3582 = T12."Enabled" ("Disabled")
        n1869 = event-data() -> ()  [unwired: 1 in, 6 out]
        n1870 = call-dynamic "Read AcquisitionA.vi"("error in (no error)"=w3615, "S4ACS_GUI in"=w3616) -> ("error out"=w3611:errorcluster, "Acquisition.lvclass"=w3614:refnum<class "Acquisition.lvclass">, "S4ACS_GUI out"=w3583:refnum<class "S4GUI.lvclass">)  [unwired: 7 in]
        n1871 = call-dynamic "Read Channel.vi"("error in (no error)"=w3611, "Acquisition in"=w3614) -> ("error out"=w3610:errorcluster, "Channel.lvclass"=w3613:refnum<class "Channel.lvclass">)  [unwired: 7 in, 1 out]
        n1872 = call-dynamic "Read Interface.vi"("error in (no error)"=w3610, "Channel in"=w3613) -> ("error out"=w3609:errorcluster, "Interface.lvclass"=w3612:refnum<class "Interface.lvclass">)  [unwired: 7 in, 1 out]
        n1873 = call-dynamic "Get CCD_Config.vi"("error in (no error)"=w3609, "Interface in"=w3612) -> ("error out"=w3606:errorcluster, "output cluster"=w3605:T31)  [unwired: 7 in, 1 out]
        n1874 = Unbundle By Name(w3605) -> ("INITIAL_LINE"=w3604:u16, "INITIAL_COLUMN"=w3603:u16, "FINAL_LINE"=w3602:u16, "FINAL_COLUMN"=w3601:u16, "VBIN"=w3600:u16, "HBIN"=w3599:u16, "PREAMP"=w3598:u8, "EM_GAIN"=w3597:u16, "READOUT_RATE"=w3596:u8, "SHUTTER_OPENING_TIME"=w3595:u16, "SHUTTER_CLOSING_TIME"=w3594:u16, "VERTICAL_SHIFT_SPEED"=w3593:u8, "READ_MODE"=w3592:u8, "VERTICAL_CLOCK_VOLTAGE"=w3591:u8, "AD_CHANNEL"=w3590:u32, "SHUTTER_MODE"=w3589:u8, "SHUTTER_TTL"=w3588:u8, "TRIGGER_MODE"=w3587:u8, "FRAME_TRANSFER"=w3586:bool, "ACQUISITION_MODE"=w3585:u8, "EM_MODE"=w3584:u8)
        n1875 = local read "Input Cluster"() -> (w3608:T8)
        n1876 = Bundle By Name(cluster=w3608, "Parameters.Image \nInitial Line"=w3604, "Parameters.Image\nInitial Column"=w3603, "Parameters.Image\nFinal Line"=w3602, "Parameters.Image\nFInal Column"=w3601, "Parameters.Vertical\nBinning"=w3600, "Parameters.Horizontal\nBinning"=w3599, "Parameters.Pre-amplification\nGain"=w3598, "Parameters.CCD\nEM Gain"=w3597, "Parameters.Readout\nRate"=w3596, "Parameters.Shutter\nOpenning Time"=w3595, "Parameters.Shutter\nClosing Time"=w3594, "Parameters.Vertical\nShift Speed"=w3593, "Parameters.Read\nMode"=w3592, "Parameters.Vertical\nClock Voltage"=w3591, "Parameters.A/D \nChannel"=w3590, "Parameters.Shutter\nMode"=w3589, "Parameters.Shutter\nTTL"=w3588, "Parameters.Trigger\nMode"=w3587, "Parameters.Frame\nTransfer"=w3586, "Parameters.Acquisition\nMode"=w3585, "Parameters.CCD \nEM Mode"=w3584) -> (w3607:T8)
        n1877 = local write "Input Cluster"(w3607) -> ()
        n1878 = property on="Set from Input ch1" class="Bool"("DisabledEnum"=w3582) -> ()  [unwired: 2 in, 2 out]
        n1879 = property on="Set from Input ch3" class="Bool"("DisabledEnum"=w3582) -> ()  [unwired: 2 in, 2 out]
        n1880 = property on="Set from Input ch2" class="Bool"("DisabledEnum"=w3582) -> ()  [unwired: 2 in, 2 out]
        n1881 = property on="Set from Input ch4" class="Bool"("DisabledEnum"=w3582) -> ()  [unwired: 2 in, 2 out]
      }
      event "Copy to Input ch2": Value Change {
        w3617 = T12."Enabled" ("Disabled")
        n1882 = event-data() -> ()  [unwired: 1 in, 6 out]
        n1883 = call "Read AcquisitionB.vi"("error in (no error)"=w3650, "S4ACS_GUI in"=w3651) -> ("error out"=w3646:errorcluster, "Acquisition.lvclass"=w3649:refnum<class "Acquisition.lvclass">, "S4ACS_GUI out"=w3618:refnum<class "S4GUI.lvclass">)  [unwired: 7 in]
        n1884 = call-dynamic "Read Channel.vi"("error in (no error)"=w3646, "Acquisition in"=w3649) -> ("error out"=w3645:errorcluster, "Channel.lvclass"=w3648:refnum<class "Channel.lvclass">)  [unwired: 7 in, 1 out]
        n1885 = call-dynamic "Read Interface.vi"("error in (no error)"=w3645, "Channel in"=w3648) -> ("error out"=w3644:errorcluster, "Interface.lvclass"=w3647:refnum<class "Interface.lvclass">)  [unwired: 7 in, 1 out]
        n1886 = call-dynamic "Get CCD_Config.vi"("error in (no error)"=w3644, "Interface in"=w3647) -> ("error out"=w3641:errorcluster, "output cluster"=w3640:T31)  [unwired: 7 in, 1 out]
        n1887 = Unbundle By Name(w3640) -> ("INITIAL_LINE"=w3639:u16, "INITIAL_COLUMN"=w3638:u16, "FINAL_LINE"=w3637:u16, "FINAL_COLUMN"=w3636:u16, "VBIN"=w3635:u16, "HBIN"=w3634:u16, "PREAMP"=w3633:u8, "EM_GAIN"=w3632:u16, "READOUT_RATE"=w3631:u8, "SHUTTER_OPENING_TIME"=w3630:u16, "SHUTTER_CLOSING_TIME"=w3629:u16, "VERTICAL_SHIFT_SPEED"=w3628:u8, "READ_MODE"=w3627:u8, "VERTICAL_CLOCK_VOLTAGE"=w3626:u8, "AD_CHANNEL"=w3625:u32, "SHUTTER_MODE"=w3624:u8, "SHUTTER_TTL"=w3623:u8, "TRIGGER_MODE"=w3622:u8, "FRAME_TRANSFER"=w3621:bool, "ACQUISITION_MODE"=w3620:u8, "EM_MODE"=w3619:u8)
        n1888 = local read "Input Cluster"() -> (w3643:T8)
        n1889 = Bundle By Name(cluster=w3643, "Parameters.Image \nInitial Line"=w3639, "Parameters.Image\nInitial Column"=w3638, "Parameters.Image\nFinal Line"=w3637, "Parameters.Image\nFInal Column"=w3636, "Parameters.Vertical\nBinning"=w3635, "Parameters.Horizontal\nBinning"=w3634, "Parameters.Pre-amplification\nGain"=w3633, "Parameters.CCD\nEM Gain"=w3632, "Parameters.Readout\nRate"=w3631, "Parameters.Shutter\nOpenning Time"=w3630, "Parameters.Shutter\nClosing Time"=w3629, "Parameters.Vertical\nShift Speed"=w3628, "Parameters.Read\nMode"=w3627, "Parameters.Vertical\nClock Voltage"=w3626, "Parameters.A/D \nChannel"=w3625, "Parameters.Shutter\nMode"=w3624, "Parameters.Shutter\nTTL"=w3623, "Parameters.Trigger\nMode"=w3622, "Parameters.Frame\nTransfer"=w3621, "Parameters.Acquisition\nMode"=w3620, "Parameters.CCD \nEM Mode"=w3619) -> (w3642:T8)
        n1890 = local write "Input Cluster"(w3642) -> ()
        n1891 = property on="Set from Input ch1" class="Bool"("DisabledEnum"=w3617) -> ()  [unwired: 2 in, 2 out]
        n1892 = property on="Set from Input ch3" class="Bool"("DisabledEnum"=w3617) -> ()  [unwired: 2 in, 2 out]
        n1893 = property on="Set from Input ch2" class="Bool"("DisabledEnum"=w3617) -> ()  [unwired: 2 in, 2 out]
        n1894 = property on="Set from Input ch4" class="Bool"("DisabledEnum"=w3617) -> ()  [unwired: 2 in, 2 out]
      }
      event "Copy to Input ch3": Value Change {
        w3652 = T12."Enabled" ("Disabled")
        n1895 = event-data() -> ()  [unwired: 1 in, 6 out]
        n1896 = call-dynamic "Read AcquisitionC.vi"("error in (no error)"=w3685, "S4ACS_GUI in"=w3686) -> ("error out"=w3681:errorcluster, "Acquisition.lvclass"=w3684:refnum<class "Acquisition.lvclass">, "S4ACS_GUI out"=w3653:refnum<class "S4GUI.lvclass">)  [unwired: 7 in]
        n1897 = call-dynamic "Read Channel.vi"("error in (no error)"=w3681, "Acquisition in"=w3684) -> ("error out"=w3680:errorcluster, "Channel.lvclass"=w3683:refnum<class "Channel.lvclass">)  [unwired: 7 in, 1 out]
        n1898 = call-dynamic "Read Interface.vi"("error in (no error)"=w3680, "Channel in"=w3683) -> ("error out"=w3679:errorcluster, "Interface.lvclass"=w3682:refnum<class "Interface.lvclass">)  [unwired: 7 in, 1 out]
        n1899 = call-dynamic "Get CCD_Config.vi"("error in (no error)"=w3679, "Interface in"=w3682) -> ("error out"=w3676:errorcluster, "output cluster"=w3675:T31)  [unwired: 7 in, 1 out]
        n1900 = Unbundle By Name(w3675) -> ("INITIAL_LINE"=w3674:u16, "INITIAL_COLUMN"=w3673:u16, "FINAL_LINE"=w3672:u16, "FINAL_COLUMN"=w3671:u16, "VBIN"=w3670:u16, "HBIN"=w3669:u16, "PREAMP"=w3668:u8, "EM_GAIN"=w3667:u16, "READOUT_RATE"=w3666:u8, "SHUTTER_OPENING_TIME"=w3665:u16, "SHUTTER_CLOSING_TIME"=w3664:u16, "VERTICAL_SHIFT_SPEED"=w3663:u8, "READ_MODE"=w3662:u8, "VERTICAL_CLOCK_VOLTAGE"=w3661:u8, "AD_CHANNEL"=w3660:u32, "SHUTTER_MODE"=w3659:u8, "SHUTTER_TTL"=w3658:u8, "TRIGGER_MODE"=w3657:u8, "FRAME_TRANSFER"=w3656:bool, "ACQUISITION_MODE"=w3655:u8, "EM_MODE"=w3654:u8)
        n1901 = local read "Input Cluster"() -> (w3678:T8)
        n1902 = Bundle By Name(cluster=w3678, "Parameters.Image \nInitial Line"=w3674, "Parameters.Image\nInitial Column"=w3673, "Parameters.Image\nFinal Line"=w3672, "Parameters.Image\nFInal Column"=w3671, "Parameters.Vertical\nBinning"=w3670, "Parameters.Horizontal\nBinning"=w3669, "Parameters.Pre-amplification\nGain"=w3668, "Parameters.CCD\nEM Gain"=w3667, "Parameters.Readout\nRate"=w3666, "Parameters.Shutter\nOpenning Time"=w3665, "Parameters.Shutter\nClosing Time"=w3664, "Parameters.Vertical\nShift Speed"=w3663, "Parameters.Read\nMode"=w3662, "Parameters.Vertical\nClock Voltage"=w3661, "Parameters.A/D \nChannel"=w3660, "Parameters.Shutter\nMode"=w3659, "Parameters.Shutter\nTTL"=w3658, "Parameters.Trigger\nMode"=w3657, "Parameters.Frame\nTransfer"=w3656, "Parameters.Acquisition\nMode"=w3655, "Parameters.CCD \nEM Mode"=w3654) -> (w3677:T8)
        n1903 = local write "Input Cluster"(w3677) -> ()
        n1904 = property on="Set from Input ch1" class="Bool"("DisabledEnum"=w3652) -> ()  [unwired: 2 in, 2 out]
        n1905 = property on="Set from Input ch3" class="Bool"("DisabledEnum"=w3652) -> ()  [unwired: 2 in, 2 out]
        n1906 = property on="Set from Input ch2" class="Bool"("DisabledEnum"=w3652) -> ()  [unwired: 2 in, 2 out]
        n1907 = property on="Set from Input ch4" class="Bool"("DisabledEnum"=w3652) -> ()  [unwired: 2 in, 2 out]
      }
      event "Copy to Input ch4": Value Change {
        w3687 = T12."Enabled" ("Disabled")
        n1908 = event-data() -> ()  [unwired: 1 in, 6 out]
        n1909 = call-dynamic "Read AcquisitionD.vi"("error in (no error)"=w3720, "S4ACS_GUI in"=w3721) -> ("error out"=w3716:errorcluster, "Acquisition.lvclass"=w3719:refnum<class "Acquisition.lvclass">, "S4ACS_GUI out"=w3688:refnum<class "S4GUI.lvclass">)  [unwired: 7 in]
        n1910 = call-dynamic "Read Channel.vi"("error in (no error)"=w3716, "Acquisition in"=w3719) -> ("error out"=w3715:errorcluster, "Channel.lvclass"=w3718:refnum<class "Channel.lvclass">)  [unwired: 7 in, 1 out]
        n1911 = call-dynamic "Read Interface.vi"("error in (no error)"=w3715, "Channel in"=w3718) -> ("error out"=w3714:errorcluster, "Interface.lvclass"=w3717:refnum<class "Interface.lvclass">)  [unwired: 7 in, 1 out]
        n1912 = call-dynamic "Get CCD_Config.vi"("error in (no error)"=w3714, "Interface in"=w3717) -> ("error out"=w3711:errorcluster, "output cluster"=w3710:T31)  [unwired: 7 in, 1 out]
        n1913 = Unbundle By Name(w3710) -> ("INITIAL_LINE"=w3709:u16, "INITIAL_COLUMN"=w3708:u16, "FINAL_LINE"=w3707:u16, "FINAL_COLUMN"=w3706:u16, "VBIN"=w3705:u16, "HBIN"=w3704:u16, "PREAMP"=w3703:u8, "EM_GAIN"=w3702:u16, "READOUT_RATE"=w3701:u8, "SHUTTER_OPENING_TIME"=w3700:u16, "SHUTTER_CLOSING_TIME"=w3699:u16, "VERTICAL_SHIFT_SPEED"=w3698:u8, "READ_MODE"=w3697:u8, "VERTICAL_CLOCK_VOLTAGE"=w3696:u8, "AD_CHANNEL"=w3695:u32, "SHUTTER_MODE"=w3694:u8, "SHUTTER_TTL"=w3693:u8, "TRIGGER_MODE"=w3692:u8, "FRAME_TRANSFER"=w3691:bool, "ACQUISITION_MODE"=w3690:u8, "EM_MODE"=w3689:u8)
        n1914 = local read "Input Cluster"() -> (w3713:T8)
        n1915 = Bundle By Name(cluster=w3713, "Parameters.Image \nInitial Line"=w3709, "Parameters.Image\nInitial Column"=w3708, "Parameters.Image\nFinal Line"=w3707, "Parameters.Image\nFInal Column"=w3706, "Parameters.Vertical\nBinning"=w3705, "Parameters.Horizontal\nBinning"=w3704, "Parameters.Pre-amplification\nGain"=w3703, "Parameters.CCD\nEM Gain"=w3702, "Parameters.Readout\nRate"=w3701, "Parameters.Shutter\nOpenning Time"=w3700, "Parameters.Shutter\nClosing Time"=w3699, "Parameters.Vertical\nShift Speed"=w3698, "Parameters.Read\nMode"=w3697, "Parameters.Vertical\nClock Voltage"=w3696, "Parameters.A/D \nChannel"=w3695, "Parameters.Shutter\nMode"=w3694, "Parameters.Shutter\nTTL"=w3693, "Parameters.Trigger\nMode"=w3692, "Parameters.Frame\nTransfer"=w3691, "Parameters.Acquisition\nMode"=w3690, "Parameters.CCD \nEM Mode"=w3689) -> (w3712:T8)
        n1916 = local write "Input Cluster"(w3712) -> ()
        n1917 = property on="Set from Input ch1" class="Bool"("DisabledEnum"=w3687) -> ()  [unwired: 2 in, 2 out]
        n1918 = property on="Set from Input ch3" class="Bool"("DisabledEnum"=w3687) -> ()  [unwired: 2 in, 2 out]
        n1919 = property on="Set from Input ch2" class="Bool"("DisabledEnum"=w3687) -> ()  [unwired: 2 in, 2 out]
        n1920 = property on="Set from Input ch4" class="Bool"("DisabledEnum"=w3687) -> ()  [unwired: 2 in, 2 out]
      }
      event "Scrollbar": Value Change {
        (unwired) 765.0 ("BarOffset")
        (unwired) 1000.0 ("BarOffset")
        n1921 = event-data() -> ()  [unwired: 1 in, 6 out]
        n1922 = disable-structure shown="Disabled" {
          disable-tunnel: w3723 -> [w3735 _]
          frame Disabled {
            # "como alterar o valor de um parametro em \"Parameter Input\""
            n1923 = Unbundle By Name(w3735) -> ("Parameters"=w3737:T5)
            n1924 = Bundle By Name(cluster=w3737, "Readout\nRate"=u8 1 ("Readout\nRate")) -> (w3734:T5)
            n1925 = Bundle By Name(cluster=w3735, "Parameters"=w3734) -> (w3733:T8)
            n1926 = local write "Input Cluster"(w3733) -> ()
          }
          frame Enabled {
          }
        }
        n1927 = property on="Scrollbar" class="Scroll (strict)"() -> ("DocMax"=w3727:dbl)  [unwired: 2 in, 2 out]
        n1928 = Unbundle(w3725) -> ("Parameters"=w3730:refnum<vi>, "Current Configuration"=w3729:refnum<vi>)
        n1929 = Subtract(x=w3727, y="Scrollbar") -> (x-y=w3731:dbl)
        n1930 = Subtract(x=w3731, y=200.0 ("BarOffset")) -> (x-y=w3728:dbl)
        n1931 = property on="Property Node" class="Clust (strict)"(reference=w3730, "Top"=w3728) -> ()  [unwired: 1 in, 2 out]
        n1932 = property on="Property Node" class="Clust (strict)"(reference=w3729, "Top"=w3728) -> ()  [unwired: 1 in, 2 out]
      }
      event "Select Positions": Value Change {
        # "Garantir que, quando em POLARIMETRIA, pelo menos WP1 esteja selecionado."
        n1933 = event-data() -> ()  [unwired: 1 in, 6 out]
        n1934 = call "Read Instrument.lvclass.vi"("error in (no error)"=w3820, "S4ACS_GUI in"=w3819) -> ("error out"=w3829:errorcluster, "Instrument.lvclass"=w3828:refnum<class "Instrument.lvclass">, "S4ACS_GUI out"=w3822:refnum<class "S4GUI.lvclass">)  [unwired: 7 in]
        n1935 = call "Read WPROT.vi"("error in (no error)"=w3829, "Instrument in"=w3828) -> ("error out"=w3821:errorcluster, "Opt_Selector.lvclass"=w3825:refnum<class "Opt_Selector.lvclass">, "Instrument out"=w3823:refnum<class "Instrument.lvclass">)  [unwired: 7 in]
        n1936 = case shown="5" "Select Positions" {
          tunnel: w3821 -> [w3863 w3876 w3889 w3902 w3915 w3924]
          tunnel: [w3861 w3874 w3887 w3898 w3913 w3922] -> w3824
          tunnel: [w3859 w3872 w3885 w3899 w3911 w3923] -> w3817
          tunnel: w3825 -> [w3864 w3877 w3890 w3903 w3916 w3925]
          tunnel: [16 8 4 8 0 0] -> w3818
          tunnel: [0.0 ("Scale.Range:Minimum") 0.0 ("Scale.Range:Minimum") 0.0 ("Scale.Range:Minimum") 0.0 ("Scale.Range:Minimum") 0.0 ("Scale.Range:Minimum") 0.0 ("Scale.Range:Minimum")] -> w3816
          tunnel: [w3856 w3869 w3882 w3895 w3908 w3921] -> w3742
          frame 0, Default {
            w3856 = u16 65535 ("sequencia")
            w3865 = TRUE ("P0")
            w3866 = TRUE ("P0")
            w3867 = TRUE ("P0")
            w3868 = TRUE ("P0")
            # "1111 1111 1111 1111 = 65.535"
            n1937 = local write "P0"(w3868) -> ()
            n1938 = local write "P1"(w3868) -> ()
            n1939 = local write "P2"(w3868) -> ()
            n1940 = local write "P3"(w3868) -> ()
            n1941 = local write "P4"(w3866) -> ()
            n1942 = local write "P5"(w3866) -> ()
            n1943 = local write "P6"(w3866) -> ()
            n1944 = local write "P7"(w3866) -> ()
            n1945 = call-dynamic "Write sequencia.vi"("error in (no error)"=w3863, "sequencia"=w3856, "Opt_Selector in"=w3864) -> ("error out"=w3860:errorcluster, "Opt_Selector out"=w3862:refnum<class "Opt_Selector.lvclass">)  [unwired: 7 in]
            n1946 = call-dynamic "Write sequencia_ant.vi"("error in (no error)"=w3860, "sequencia_ant"=w3856, "Opt_Selector in"=w3862) -> ("error out"=w3859:errorcluster, "Opt_Selector out"=w3861:refnum<class "Opt_Selector.lvclass">)  [unwired: 7 in]
            n1947 = local write "P8"(w3867) -> ()
            n1948 = local write "P9"(w3867) -> ()
            n1949 = local write "P10"(w3867) -> ()
            n1950 = local write "P11"(w3867) -> ()
            n1951 = local write "P12"(w3865) -> ()
            n1952 = local write "P13"(w3865) -> ()
            n1953 = local write "P14"(w3865) -> ()
            n1954 = local write "P15"(w3865) -> ()
          }
          frame 1 {
            w3869 = u16 255 ("sequencia")
            w3878 = FALSE ("P0")
            w3879 = TRUE ("P0")
            w3880 = FALSE ("P0")
            w3881 = TRUE ("P0")
            # "0000 0000 1111 1111 = 255"
            n1955 = local write "P0"(w3881) -> ()
            n1956 = local write "P1"(w3881) -> ()
            n1957 = local write "P2"(w3881) -> ()
            n1958 = local write "P3"(w3881) -> ()
            n1959 = local write "P4"(w3879) -> ()
            n1960 = local write "P5"(w3879) -> ()
            n1961 = local write "P6"(w3879) -> ()
            n1962 = local write "P7"(w3879) -> ()
            n1963 = call-dynamic "Write sequencia.vi"("error in (no error)"=w3876, "sequencia"=w3869, "Opt_Selector in"=w3877) -> ("error out"=w3873:errorcluster, "Opt_Selector out"=w3875:refnum<class "Opt_Selector.lvclass">)  [unwired: 7 in]
            n1964 = local write "P8"(w3880) -> ()
            n1965 = local write "P9"(w3880) -> ()
            n1966 = local write "P10"(w3880) -> ()
            n1967 = local write "P11"(w3880) -> ()
            n1968 = local write "P12"(w3878) -> ()
            n1969 = local write "P13"(w3878) -> ()
            n1970 = local write "P14"(w3878) -> ()
